vi "Check Channel Overload.vi"(0 "device session in":refnum<class "Device Session.lvclass">, 11 "error in":errorcluster) -> (4 "device session out":refnum<class "Device Session.lvclass">, 15 "error out":errorcluster)   [LabVIEW 2015, in "Device Session.lvclass"]
doc: "Checks all input channels on the device for overload conditions, and returns an error if an overload has occurred on any channel.\n\n<B>Input Parameters</B>\n\n<B>device session in</B> is a reference to the session containing sessions to all instrument design libraries used in this sample project. This parameter is obtained from the 'Open Session' VI.\n\n<B>error in</B> describes error conditions that occur before this node runs. This input provides standard 'error in' functionality.\n\n<B>Output Parameters</B>\n\n<B>device session out</B> passes a reference to the session to the next VI.\n\n<B>error out</B> contains error information. This output provides standard 'error out' functionality."
uses:
  Device Session.lvclass
  Device Session.lvclass/Device Session.ctl
  <instrlib>/HSAI-RIO/Config/Interface/v1/Host/niHSAI Config v1 Host.lvclass
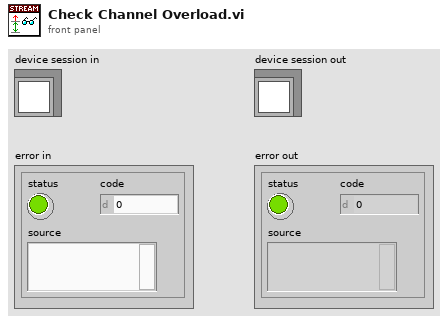
[diagram p1: front panel]
types:
  T1 = typedef "Device Session.lvclass/Device Session Object.ctl" = cluster{"ni5171R FPGA Reference":T2, "niHSAI config":refnum<class "niHSAI Config v1 Host.lvclass">, "configured scaling coefficients":cluster{"gain":dbl, "offset":dbl}[], "number of channels to stream":u8, "selected acq channels":bool[], "number of channels":u32, "actual channel configuration":T3[], "configured channels":bool[], "sample clock rate (Hz)":dbl}
  T2 = typedef "Device Session.lvclass/FPGA Refnum.ctl" = refnum<k20>
  T3 = typedef "niHSAI Types v1 Host.lvlib/Channel Configuration.ctl" = cluster{"channel":u32, "coupling":T4, "impedance":T5, "bandwidth":T6, "vertical range":dbl, "vertical offset":dbl}
  T4 = typedef "niHSAI Types v1 Host.lvlib/Coupling.ctl" = enum8{"Default", "DC", "AC"}
  T5 = typedef "niHSAI Types v1 Host.lvlib/Impedance.ctl" = enum8{"Default", "1 mega ohm", "50 ohm"}
  T6 = typedef "niHSAI Types v1 Host.lvlib/Bandwidth.ctl" = enum8{"Default", "Full Bandwidth", "Anti-alias Filter"}
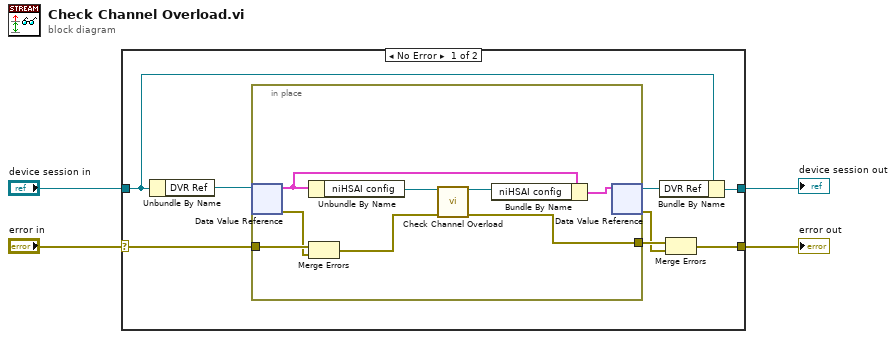
[diagram p0: block diagram]
diagram:
  n1 = case shown="No Error" "error in" {
    selector: "error in" -> [w11 w21]
    tunnel: "device session in" -> [w7 w22]
    tunnel: [w5 w22] -> w2
    tunnel: [w10 w21] -> w1
    frame No Error {
      n2 = Unbundle By Name(w7) -> ("DVR Ref"=w12:refnum<data-value>)
      n3 = in-place {
        in-place-border: w11 -> [w20]
        in-place-border: [w13] -> w9
        n4 = in-place-dvr #1(w12) -> (w16:T1, w19:errorcluster)
        n5 = Unbundle By Name(w16) -> ("niHSAI config"=w18:refnum<class "niHSAI Config v1 Host.lvclass">)
        n6 = Merge Errors(w20, w19) -> (w17:errorcluster)
        n7 = call-dynamic "Check Channel Overload.vi"("session in"=w18, "error in"=w17) -> ("session out"=w15:refnum<class "niHSAI Config v1 Host.lvclass">, "error out"=w13:errorcluster)  [unwired: 11 in, 1 out]
        n8 = Bundle By Name(cluster=w16, "niHSAI config"=w15) -> (w14:T1)
        n9 = in-place-dvr #1(w14) -> (w6:refnum<data-value>, w8:errorcluster)
      }
      n10 = Bundle By Name(cluster=w7, "DVR Ref"=w6) -> (w5:refnum<class "Device Session.lvclass">)
      n11 = Merge Errors(w9, w8) -> (w10:errorcluster)
    }
    frame Error {
    }
  }
  "error out" <- w1
  "device session out" <- w2
